vi "Set IT.vi"(10 "IT":i32, 11 "handle":i32) -> (2 "function return":i32, 3 "handle out":i32)   [LabVIEW 2022 SP3]
doc: "BOOL H11890API __stdcall H11890SetIT(HANDLE handle,DWORD IT);"
uses:
  H11890api.dll
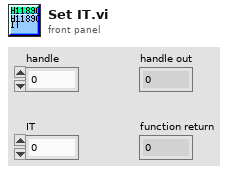
[diagram p1: front panel]
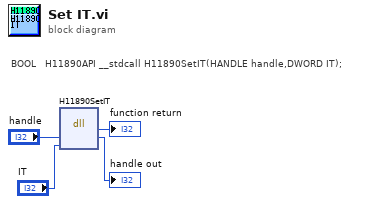
[diagram p0: block diagram]
diagram:
  # "BOOL\t\t\tH11890API\t__stdcall H11890SetIT(HANDLE handle,DWORD IT);"
  n1 = dll-call lib="H:/.shortcut-targets-by-id/1riZacJd_1_jmKfGgrjDuP7KcecvMS3i2/Xiao research group/Programs/LabviewControlPrograms/scanner_stepper_and_mapping/PMT_mapping/H11890api.dll" fn="H11890SetIT"("handle"="handle", "IT"="IT") -> ("Return"=→"function return":i32, "handle"=→"handle out":i32)  [unwired: 4 in, 2 out]
